vi "Get Curr and Volt.vi"(0 "PS Test in":refnum<class "PS Test.lvclass">, 11 "error in (no error)":errorcluster) -> (4 "PS Test out":refnum<class "PS Test.lvclass">, 6 "Voltage":dbl, 8 "Current":dbl, 10 "Output?":bool, 15 "error out":errorcluster)   [LabVIEW 2021, in "PS.lvlib" / "PS Test.lvclass"]
uses:
  PS Test.lvclass
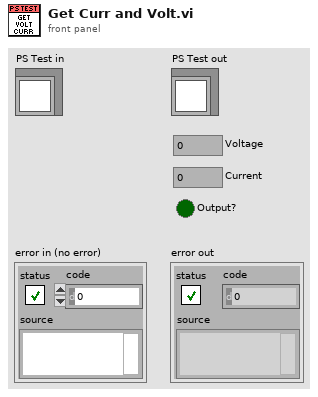
[diagram p1: front panel]
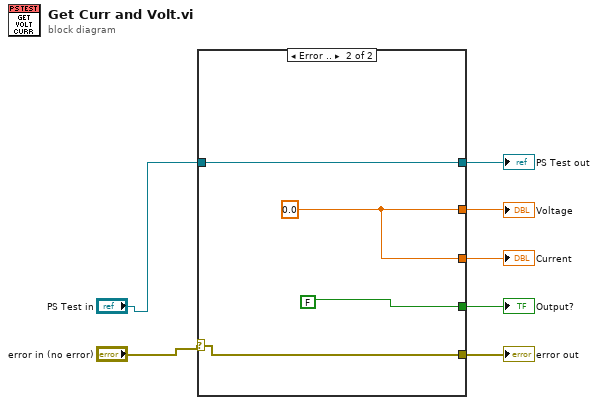
[diagram p0: block diagram]
diagram:
  n1 = case shown="Error .." "error in (no error)" {
    selector: "error in (no error)" -> [w9 w12]
    tunnel: [w9 w12] -> w6
    tunnel: [w8 w13] -> w5
    tunnel: "PS Test in" -> [w8 w13]
    tunnel: [_ w11] -> w3
    tunnel: [_ w11] -> w2
    tunnel: [_ FALSE] -> w1
    frame No Error {
    }
    frame Error {
      w11 = 0.0
    }
  }
  "error out" <- w6
  "PS Test out" <- w5
  "Current" <- w2
  "Voltage" <- w3
  "Output?" <- w1
